vi "linearfit_new.vi"(8 "array 2":dbl[](array[numeric]), 9 "index 2":i32, 10 "index":i32, 11 "array":dbl[](array[numeric])) -> (1 "intercept":dbl, 2 "slope":dbl)   [LabVIEW 2014]
uses:
  <vilib>/Analysis/baseanly.llb/Mean (DBL).vi
  <vilib>/Analysis/NI_AALBase.lvlib
  <vilib>/Analysis/NI_AALPro.lvlib
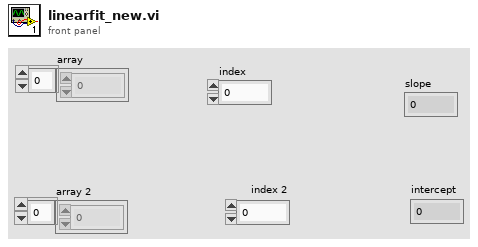
[diagram p1: front panel]
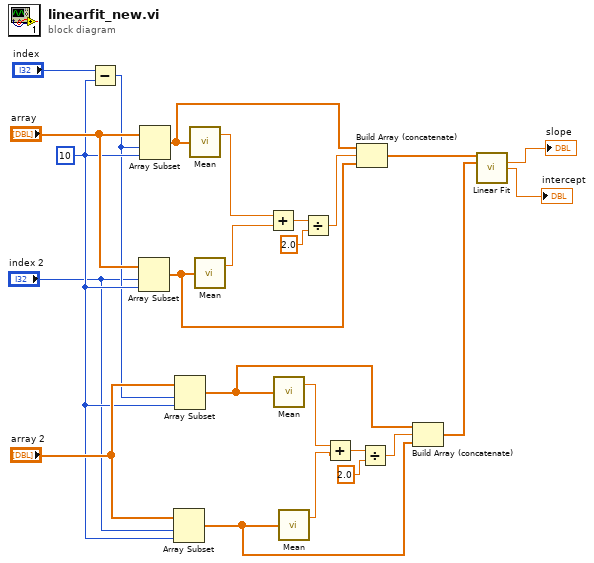
[diagram p0: block diagram]
diagram:
  w10 = 10 ("length")
  n1 = Subtract(x="index", y=w10) -> (x-y=w9:i32)
  n2 = Array Subset(array="array", index="index 2", length=w10) -> (w17:dbl[])
  n3 = Array Subset(array="array", index=w9, length=w10) -> (w19:dbl[])
  n4 = Array Subset(array="array 2", index="index 2", length=w10) -> (w1:dbl[])
  n5 = Array Subset(array="array 2", index=w9, length=w10) -> (w3:dbl[])
  n6 = call-poly <vilib>:"Mean.vi"("X"=w19) -> ("mean"=w23:dbl)  [unwired: 1 out]
  n7 = call-poly <vilib>:"Mean.vi"("X"=w17) -> ("mean"=w22:dbl)  [unwired: 1 out]
  n8 = Add(x=w23, y=w22) -> (x+y=w21:dbl)
  n9 = call-poly <vilib>:"Mean.vi"("X"=w3) -> ("mean"=w5:dbl)  [unwired: 1 out]
  n10 = call-poly <vilib>:"Mean.vi"("X"=w1) -> ("mean"=w4:dbl)  [unwired: 1 out]
  n11 = Divide(x=w21, y=2.0) -> (x/y=w18:dbl)
  n12 = Add(x=w5, y=w4) -> (x+y=w7:dbl)
  n13 = Build Array (concatenate)(w19, w18, w17) -> (w16:dbl[])
  n14 = Divide(x=w7, y=2.0) -> (x/y=w2:dbl)
  n15 = Build Array (concatenate)(w3, w2, w1) -> (w12:dbl[])
  n16 = call <vilib>:"Linear Fit.vi"("Y"=w16, "X"=w12) -> ("slope"=→"slope":dbl, "intercept"=→"intercept":dbl)  [unwired: 9 in, 3 out]
